vi "subindice mesa.vi"(11 "NewVal":T1) -> (3 "Numeric":dbl)   [LabVIEW 2015]
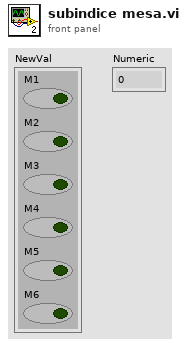
[diagram p1: front panel]
types:
  T1 = cluster{"M1":bool, "M2":bool, "M3":bool, "M4":bool, "M5":bool, "M6":bool}
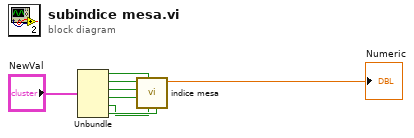
[diagram p0: block diagram]
diagram:
  n1 = Unbundle("NewVal") -> ("M1"=w1:bool, "M2"=w2:bool, "M3"=w3:bool, "M4"=w4:bool, "M5"=w5:bool, "M6"=w6:bool)
  n2 = call "indice mesa.vi"("M6"=w6, "M5"=w5, "M1"=w1, "M4"=w4, "M3"=w3, "M2"=w2) -> ("Numeric"=→"Numeric":dbl)  [unwired: 5 in]
